vi "Update Tag.vi"(8 "error in (no error)":errorcluster, 9 "Child Text":string[][](array[string]), 10 "Tag":string[](array[string]), 11 "Tag Tree In":refnum<class "Tag Tree.lvclass">) -> (0 "error out":errorcluster, 3 "Tag Tree Out":refnum<class "Tag Tree.lvclass">)   [LabVIEW 2020, in "Tree Helpers.lvlib" / "Tag Tree.lvclass"]
uses:
  Tag Tree.lvclass
  Tag Tree.lvclass/Tag Tree.ctl
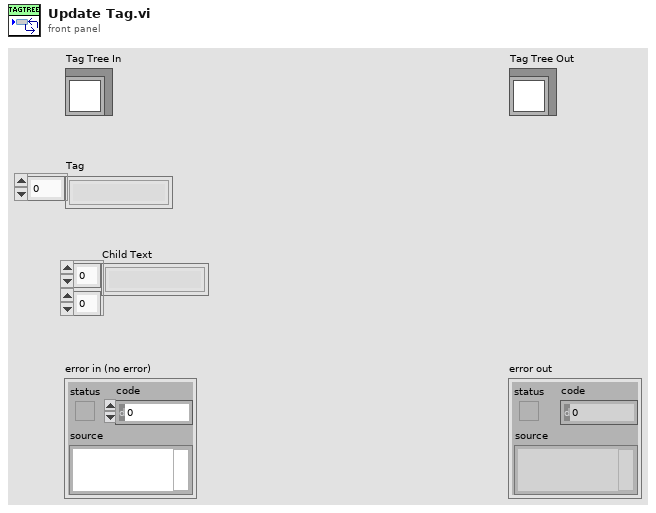
[diagram p1: front panel]
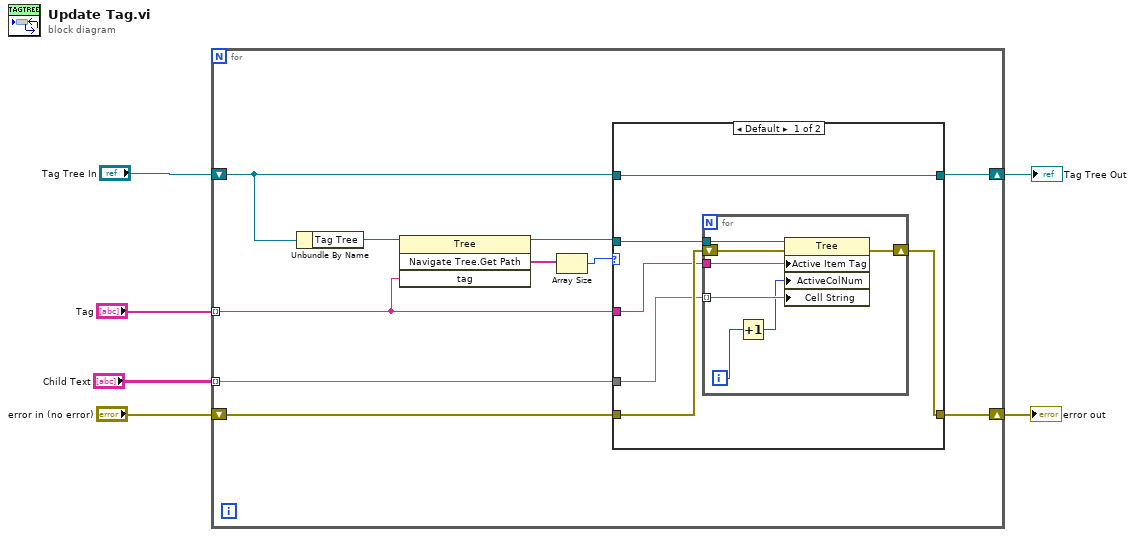
[diagram p0: block diagram]
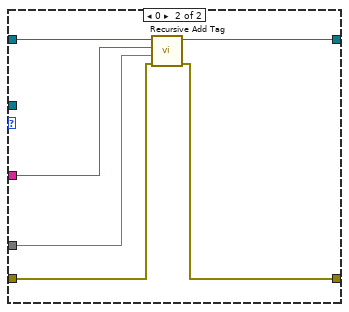
[diagram p2: hidden frame]
diagram:
  n1 = for {
    tunnel: "Tag" -> [w15] mode=indexing
    tunnel: "Child Text" -> [w12] mode=indexing
    shift-right: [w14] -> w4
    shift-left: "Tag Tree In" -> [w16]
    shift-right: [w13] -> w3
    shift-left: "error in (no error)" -> [w11]
    n2 = Unbundle By Name(w16) -> ("Tag Tree"=w10:refnum<vi>)
    n3 = invoke on="Invoke Node" class="Tree" method="Navigate Tree.Get Path"(reference=w10, "tag"=w15) -> (reference out=w9:refnum<vi>, "Navigate Tree:Get Path"=w7:string[])  [unwired: 2 in, 2 out]
    n4 = Array Size(array=w7) -> (size(s)=w8:i32)
    n5 = case shown="Default" w8 {
      tunnel: [w22 w30] -> w13
      tunnel: w11 -> [w21 w31]
      tunnel: w12 -> [w20 w32]
      tunnel: w9 -> [w19 _]
      tunnel: w15 -> [w18 w33]
      tunnel: w16 -> [w17 w35]
      tunnel: [w17 w34] -> w14
      frame Default {
        n6 = for {
          tunnel: w19 -> [w29]
          tunnel: w18 -> [w26]
          shift-right: [w28] -> w22
          shift-left: w21 -> [w27]
          tunnel: w20 -> [w25] mode=indexing
          i -> [w24]
          n7 = Increment(x=w24) -> (x+1=w23:i32)
          n8 = property on="Property Node" class="Tree"(reference=w29, error in=w27, "Active Item Tag"=w26, "ActiveColNum"=w23, "Cell String"=w25) -> (error out=w28:errorcluster)  [unwired: 1 out]
        }
      }
      frame 0 {
        n9 = call "Recursive Add Tag.vi"("error in (no error)"=w31, "Child Text"=w32, "Tag"=w33, "Tag Tree In"=w35) -> ("error out"=w30:errorcluster, "Tag Tree Out"=w34:refnum<class "Tag Tree.lvclass">)  [unwired: 6 in]
      }
    }
  }
  "error out" <- w3
  "Tag Tree Out" <- w4
